vi "ReadTirf.vi"(4 "Averages":i32=1 min=1) -> ()   [LabVIEW 2014]
uses:
  TIRF-Lock/TIRF-Lock.dll
panel:
  out "error out":errorcluster
  in  "stop":bool
  out "SUM":dbl
  out "Y":dbl
  out "X":dbl
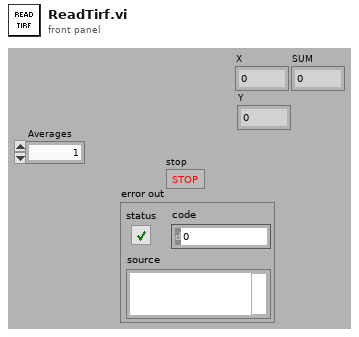
[diagram p1: front panel]
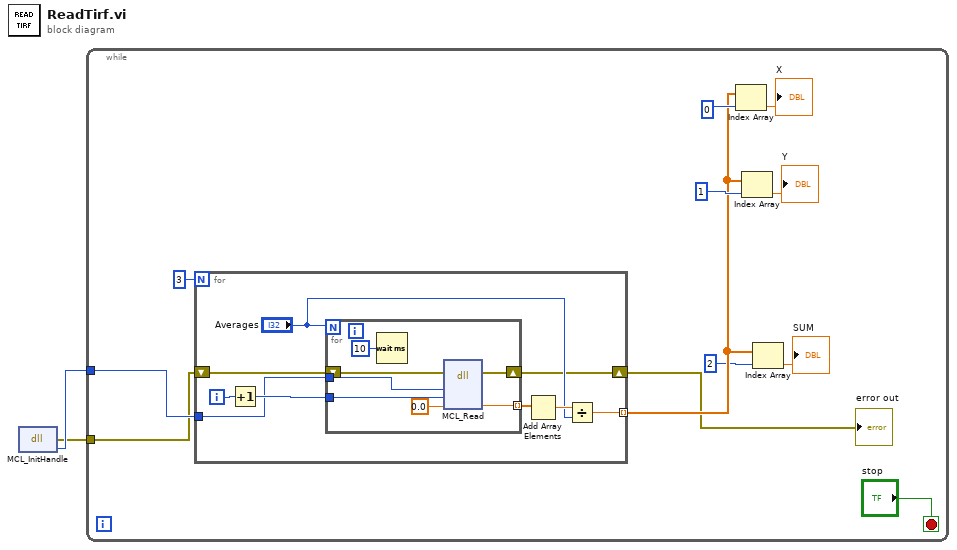
[diagram p0: block diagram]
diagram:
  n1 = dll-call lib="C:/Users/Lambda2/Desktop/Testing/TIRF-Lock/TIRF-Lock.dll" fn="MCL_InitHandle"() -> (error out=w1:errorcluster, "handle"=w2:i32)  [unwired: 3 in, 1 out]
  n2 = while {
    tunnel: w2 -> [w5]
    tunnel: w1 -> [w3]
    stop <- "stop" stop-if-true
    n3 = for {
      N: 3 -> [_]
      tunnel: [w20] -> w12 mode=indexing
      tunnel: w5 -> [w17]
      shift-right: [w16] -> w4
      shift-left: w3 -> [w15]
      i -> [w18]
      n4 = Increment(x=w18) -> (x+1=w19:i32)
      n5 = for {
        N: "Averages" -> [_]
        tunnel: w17 -> [w27]
        tunnel: [w29] -> w22 mode=indexing
        tunnel: w19 -> [w28]
        shift-right: [w25] -> w16
        shift-left: w15 -> [w24]
        n6 = Wait (ms)(milliseconds to wait=10) -> ()  [unwired: 1 out]
        n7 = dll-call lib="C:/Users/Lambda2/Desktop/Testing/TIRF-Lock/TIRF-Lock.dll" fn="MCL_Read" label="tirf read"(error in=w24, "handle"=w27, "axis"=w28, "readValue"=0.0) -> (error out=w25:errorcluster, "readValue"=w29:dbl)  [unwired: 4 in, 2 out]
      }
      n8 = Add Array Elements(numeric array=w22) -> (sum=w23:dbl)
      n9 = Divide(x=w23, y="Averages") -> (x/y=w20:dbl)
    }
    "error out" <- w4
    n10 = Index Array(array=w12, index=0) -> (element=→"X":dbl)
    n11 = Index Array(array=w12, index=1) -> (element=→"Y":dbl)
    n12 = Index Array(array=w12, index=2) -> (element=→"SUM":dbl)
  }
